vi "Aerosol Opened.vi"(8 "error in (no error)":errorcluster, 11 "Main.lvlib:Main.lvclass":refnum<class "Main.lvclass">) -> (0 "error out":errorcluster, 3 "Main.lvlib:Main.lvclass 2":refnum<class "Main.lvclass">)   [LabVIEW 2018, in "Main.lvlib" / "Main.lvclass"]
uses:
  Main.lvclass
  Main.lvclass/Main.ctl
  Feeder Actor/Feeder Messages/Set Feeder Msg/Set Feeder Msg.lvclass/Set Feeder Msg.ctl
  <vilib>/ActorFramework/Message Enqueuer/Message Enqueuer.lvclass/Message Enqueuer.ctl
  <vilib>/ActorFramework/Message Enqueuer/Enqueue.vi
  Feeder Actor/Feeder Messages/Set Feeder Msg/Set Feeder Msg.lvclass
  C:/Program Files/National Instruments/LabVIEW 2018/vi.lib/ActorFramework/Message/Message.lvclass
  <vilib>/ActorFramework/Message Priority Queue/Priority Enqueue.vi
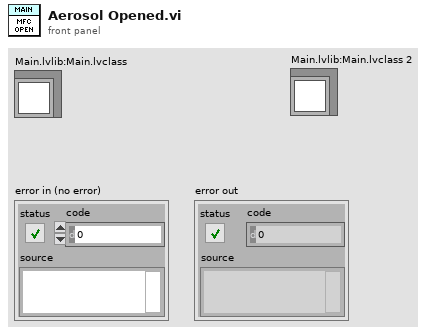
[diagram p1: front panel]
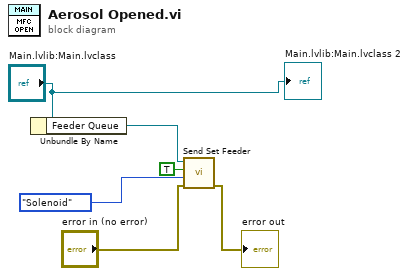
[diagram p0: block diagram]
diagram:
  n1 = Unbundle By Name("Main.lvlib:Main.lvclass") -> ("Feeder Queue"=w6:refnum<class "Message Enqueuer.lvclass">)
  n2 = call "Send Set Feeder.vi"("error in (no error)"="error in (no error)", "Component"=enum16{"All", "Mixer", "Screw", "Solenoid"}."Solenoid", "State"=TRUE, "Message Enqueuer in"=w6) -> ("error out"=→"error out":errorcluster)  [unwired: 6 in, 1 out]
  "Main.lvlib:Main.lvclass 2" <- "Main.lvlib:Main.lvclass"
